vi "AFG3352X.set frequency.vi"(0 "i ref in":refnum<vi>, 1 "Channel (1: 1)":i32(ring)=1 items=["1"=1, "2"=2], 2 "frequency [Hz]":dbl, 3 "ms timeout (10000)":i32=10000, 5 "error in (no error)":errorcluster) -> (14 "i ref out":refnum<vi>, 17 "timed out":bool, 19 "error out":errorcluster)   [LabVIEW 2014, in "AFG3352X.lvlib"]
doc: "Sets the frequency at my device."
uses:
  AFG3352X.lvlib
  CS_Core/CSApplicationBaseClasses/AFGBase/AFGBase.serviceType.ctl
  CS_Core/CSApplicationBaseClasses/AFGBase/AFGBase.directionType.ctl
  CSlibraries/UtilityLib/UtilityLib.valueStatus.ctl
  CS_Core/CSApplicationBaseClasses/DeviceBase/DeviceBase.lvlib
  CS_Core/CSApplicationBaseClasses/AFGBase/AFGBase.lvlib
  CSlibraries/UtilityLib/UtilityLib.lvlib
  instr.lib/Agilent 3352X Series/Agilent 3352X Series.lvlib
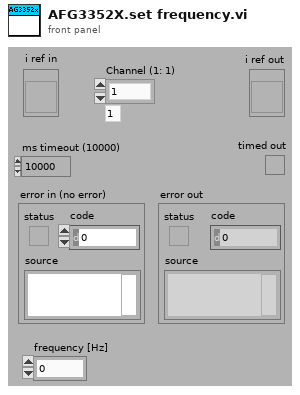
[diagram p1: front panel]
types:
  T1 = typedef "UtilityLib.lvlib/UtilityLib.valueStatus.ctl" = enum16{"no info available", "stand by/off", "on", "warning", "alarm/malfunction", "not implemented", "user action required", "important information", "system default", "control default", "indicator default", "button default"}
  T2 = typedef "AFGBase.lvlib/AFGBase.directionType.ctl" = enum16{"unknown", "update actual value", "update nominal value", "update both"}
  T3 = typedef "AFGBase.lvlib/AFGBase.serviceType.ctl" = enum16{"frequency", "amplitude", "phase", "DCOffset", "enableOutput", "trigger", "waveformType"}
  T4 = typedef "AFG3352X.lvlib/AFG3352X.i attribute.ctl" = cluster{"Act2ndValues":cluster{"frequency":dbl, "amplitude":dbl, "phase":dbl, "DCOffset":dbl, "waveformType":T5, "enableOutput":bool, "trigger":i16[], "serviceIDs":cluster{"frequencyID":i32, "amplitudeID":i32, "phaseID":i32, "DCOffsetID":i32, "waveformTypeID":i32, "enableOutputID":i32, "triggerID":i32}, "waveform":cluster{"data":waveform(dbl), "gain":dbl, "offset":dbl, "repetitionRate":dbl, "sampleRate":dbl}}, "Nom2ndValues":cluster{"frequency":dbl, "amplitude":dbl, "phase":dbl, "DCOffset":dbl, "waveformType":T5, "enableOutput":bool, "trigger":i16[], "serviceIDs":cluster{"frequencyID":i32, "amplitudeID":i32, "phaseID":i32, "DCOffsetID":i32, "waveformTypeID":i32, "enableOutputID":i32, "triggerID":i32}, "waveform":cluster{"data":waveform(dbl), "gain":dbl, "offset":dbl, "repetitionRate":dbl, "sampleRate":dbl}}, "DefaultChannel":i32, "ActAddValues":cluster{"Mode1":u16, "serviceIDs":cluster{"Mode1ID":i32, "Mode2ID":i32, "Burst1ID":i32, "Burst2ID":i32}, "Mode2":u16, "Burst1":i32, "Burst2":i32}, "NomAddValues":cluster{"Mode1":u16, "serviceIDs":cluster{"Mode1ID":i32, "Mode2ID":i32, "Burst1ID":i32, "Burst2ID":i32}, "Mode2 2":u16, "Burst1":i32, "Burst2":i32}, "enableBurstMode":bool}
  T5 = typedef "AFGBase.lvlib/AFGBase.waveformType.ctl" = enum16{"sine", "square", "ramp", "pulse", "noise", "DC", "arbitrary", "triangle", "ramp_up", "ramp_down", "amplitude modulation"}
  T6 = typedef "AFGBase.lvlib/AFGBase.i attribute.ctl" = cluster{"actValues":T7, "nomValues":T7}
  T7 = typedef "AFGBase.lvlib/AFGBase.parameters.ctl" = cluster{"frequency":dbl, "amplitude":dbl, "phase":dbl, "DCOffset":dbl, "waveformType":T5, "enableOutput":bool, "trigger":i16[], "serviceIDs":cluster{"frequencyID":i32, "amplitudeID":i32, "phaseID":i32, "DCOffsetID":i32, "waveformTypeID":i32, "enableOutputID":i32, "triggerID":i32}, "waveform":cluster{"data":waveform(dbl), "gain":dbl, "offset":dbl, "repetitionRate":dbl, "sampleRate":dbl}}
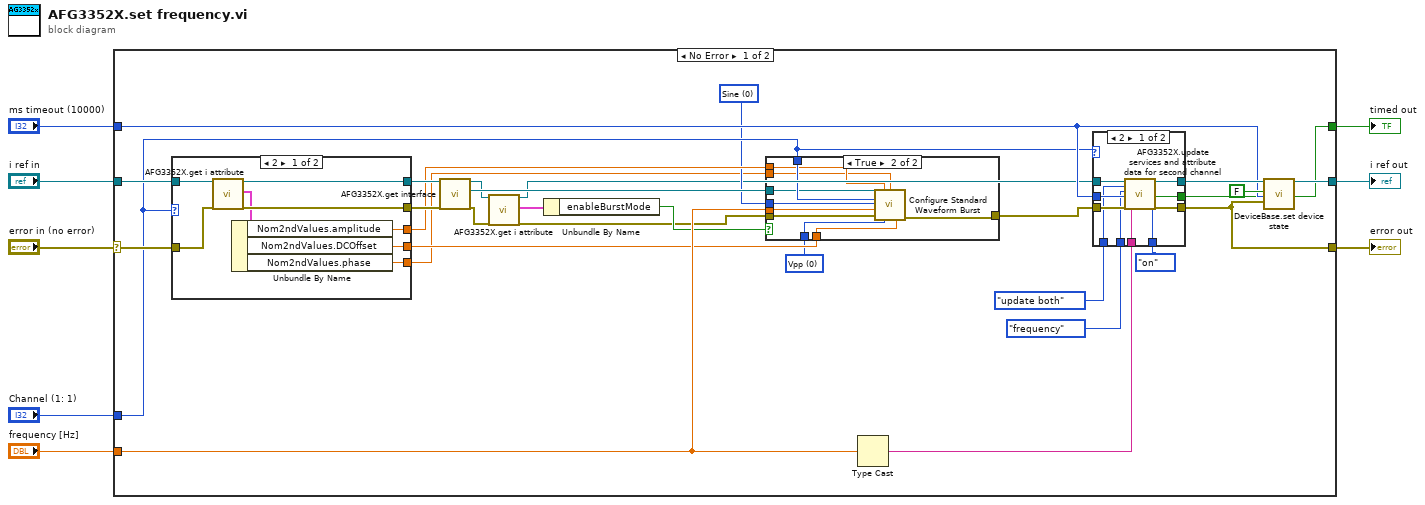
[diagram p0: block diagram]
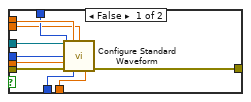
[diagram p2: hidden frame]
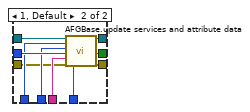
[diagram p3: hidden frame]
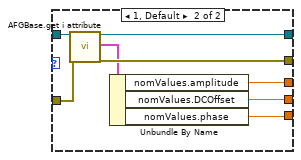
[diagram p4: hidden frame]
diagram:
  n1 = case shown="No Error" "error in (no error)" {
    selector: "error in (no error)" -> [w26 w94]
    tunnel: [w37 w95] -> w8
    tunnel: "ms timeout (10000)" -> [w33 _]
    tunnel: "i ref in" -> [w27 w95]
    tunnel: [w34 w94] -> w4
    tunnel: "frequency [Hz]" -> [w20 _]
    tunnel: [w22 _] -> w2
    tunnel: "Channel (1: 1)" -> [w17 _]
    frame No Error {
      w16 = 0 items=["Sine"=0, "Square"=1, "Ramp"=2, "Noise"=3, "DC"=4, "Triangle"=5, "Pulse"=6, "Sinc"=11, "D-Lorentz"=12, "Gaussian"=13, "Expo Fall"=14, "Expo Rise"=15, "Haversine"=16] ("Waveform Function (0: Sine)")
      w18 = u16 0 items=["Vpp", "Vrms", "dB"] ("Unit (0: Vpp)")
      n2 = case shown="2" w17 {
        tunnel: w27 -> [w85 w93]
        tunnel: w26 -> [w84 w92]
        tunnel: [w83 w91] -> w25
        tunnel: [w82 w90] -> w24
        tunnel: [w80 w88] -> w21
        tunnel: [w79 w87] -> w19
        tunnel: [w78 w86] -> w15
        frame 2 {
          n3 = call "AFG3352X.get i attribute.vi"("i ref in"=w85, "error in (no error)"=w84) -> ("i ref out"=w82:refnum<vi>, "i attribute"=w81:T4, "error out"=w83:errorcluster)  [unwired: 15 in]
          n4 = Unbundle By Name(w81) -> ("Nom2ndValues.amplitude"=w80:dbl, "Nom2ndValues.DCOffset"=w79:dbl, "Nom2ndValues.phase"=w78:dbl)
        }
        frame 1, Default {
          n5 = call "AFGBase.get i attribute.vi"("i ref in"=w93, "error in (no error)"=w92) -> ("i ref out"=w90:refnum<vi>, "i attribute"=w89:T6, "error out"=w91:errorcluster)  [unwired: 15 in]
          n6 = Unbundle By Name(w89) -> ("nomValues.amplitude"=w88:dbl, "nomValues.DCOffset"=w87:dbl, "nomValues.phase"=w86:dbl)
        }
      }
      n7 = call "AFG3352X.get interface.vi"("i ref in"=w24, "error in (no error)"=w25) -> ("i ref out"=w12:refnum<vi>, "interface"=w28:refnum<visa-resource-name>, "error out"=w10:errorcluster)  [unwired: 15 in]
      n8 = call "AFG3352X.get i attribute.vi"("i ref in"=w12, "error in (no error)"=w10) -> ("i ref out"=w11:refnum<vi>, "i attribute"=w14:T4, "error out"=w9:errorcluster)  [unwired: 15 in]
      n9 = Unbundle By Name(w14) -> ("enableBurstMode"=w13:bool)
      n10 = case shown="True" w13 {
        tunnel: w28 -> [w47 w55]
        tunnel: w9 -> [w46 w52]
        tunnel: [w45 w51] -> w23
        tunnel: w21 -> [w44 w56]
        tunnel: w20 -> [w43 w53]
        tunnel: w19 -> [w42 w50]
        tunnel: w18 -> [w41 w49]
        tunnel: w17 -> [w40 w57]
        tunnel: w16 -> [w39 w54]
        tunnel: w15 -> [w38 w48]
        frame False {
          n11 = call "Configure Standard Waveform.vi"("VISA resource name"=w47, "Amplitude (0.1 Vpp)"=w44, "Phase Angle (0 Degree)"=w38, "Channel (1: 1)"=w40, "Waveform Function (0: Sine)"=w39, "Frequency/Sample Rate/Bandwidth (1000 Hz)"=w43, "error in (no error)"=w46, "Amplitude Unit (0: Vpp)"=w41, "DC Offset (0 V)"=w42) -> ("error out"=w45:errorcluster)  [unwired: 5 in, 1 out]
        }
        frame True {
          n12 = call "Configure Standard Waveform Burst.vi"("VISA resource name"=w55, "Amplitude (0.1 Vpp)"=w56, "Phase Angle (0 Degree)"=w48, "Channel (1: 1)"=w57, "Waveform Function (0: Sine)"=w54, "Frequency/Sample Rate/Bandwidth (1000 Hz)"=w53, "error in (no error)"=w52, "Amplitude Unit (0: Vpp)"=w49, "DC Offset (0 V)"=w50) -> ("error out"=w51:errorcluster)  [unwired: 5 in, 1 out]
        }
      }
      n13 = Type Cast(x=w20) -> (*(type *) &x=w31:string)  [unwired: 1 in]
      n14 = case shown="2" w17 {
        tunnel: [w64 w77] -> w35
        tunnel: [w65 w76] -> w34
        tunnel: w33 -> [w60 w75]
        tunnel: AFGBase.serviceType."frequency" ("service") -> [w59 w74]
        tunnel: w31 -> [w61 w73]
        tunnel: AFGBase.directionType."update both" ("direction") -> [w58 w72]
        tunnel: UtilityLib.valueStatus."on" ("quality") -> [w62 w71]
        tunnel: w23 -> [w66 w70]
        tunnel: w11 -> [w67 w69]
        tunnel: [w63 w68] -> w22
        frame 2 {
          n15 = call "AFG3352X.update services and attribute data for second channel.vi"("i ref in"=w67, "direction"=w58, "service"=w59, "ms timeout (10000)"=w60, "value"=w61, "error in (no error)"=w66, "quality"=w62) -> ("i ref out"=w64:refnum<vi>, "timed out"=w63:bool, "error out"=w65:errorcluster)  [unwired: 10 in]
        }
        frame 1, Default {
          n16 = call "AFGBase.update services and attribute data.vi"("i ref in"=w69, "direction"=w72, "service"=w74, "ms timeout (10000)"=w75, "value"=w73, "error in (no error)"=w70, "quality"=w71) -> ("i ref out"=w77:refnum<vi>, "timed out"=w68:bool, "error out"=w76:errorcluster)  [unwired: 10 in]
        }
      }
      n17 = call "DeviceBase.set device state.vi"("i ref in"=w35, "implicit"=FALSE, "ms timeout (10000)"=w33, "device error"=w34) -> ("i ref out"=w37:refnum<vi>)  [unwired: 13 in, 2 out]
    }
    frame Error {
    }
  }
  "error out" <- w4
  "i ref out" <- w8
  "timed out" <- w2
